vi "Sweep SL WL.vi"(8 "error in (no error)":errorcluster, 9 "Sweep outfile":path, 10 "addr":i32, 11 "instrument handle":refnum<k15>) -> (0 "error out":errorcluster, 1 "final current (A)":dbl, 2 "final resistance (ohm)":dbl, 3 "instrument handle out":refnum<k15>)   [LabVIEW 2018]
uses:
  <vilib>/Utility/file.llb/Write Delimited Spreadsheet (DBL).vi
panel:
  out "i":i32
  out "PW":i32
  out "SL voltage (V)":dbl
  out "WL voltage (V)":dbl
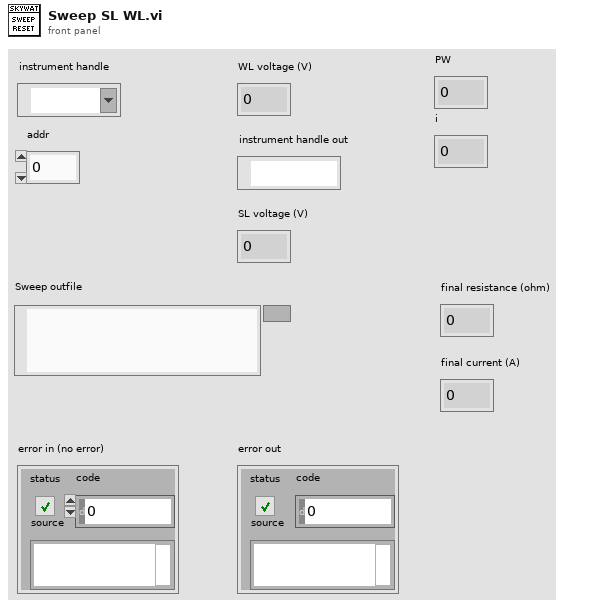
[diagram p1: front panel]
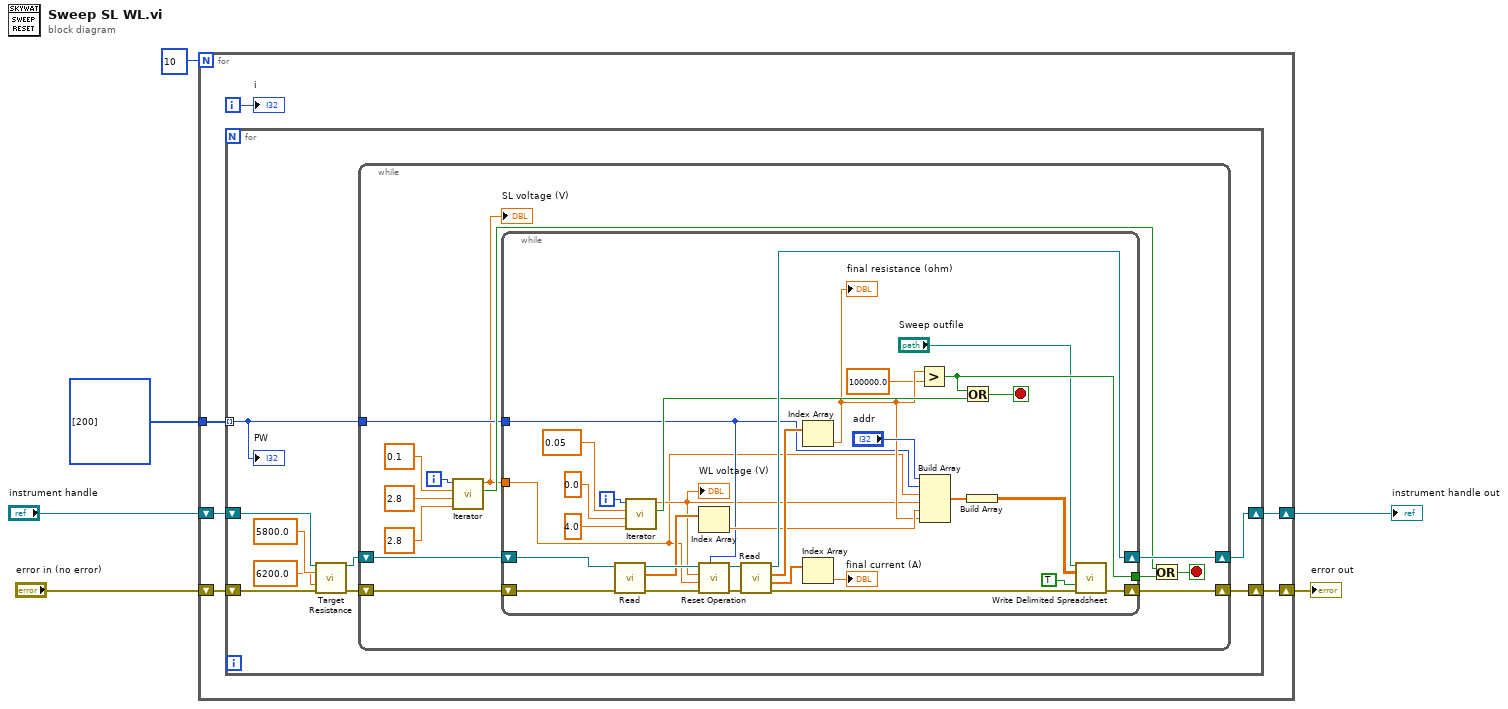
[diagram p0: block diagram]
diagram:
  n1 = for {
    N: 10 -> [_]
    tunnel: i32[] [200] -> [w8]
    shift-right: [w12] -> w6
    shift-left: "instrument handle" -> [w11]
    shift-right: [w9] -> w3
    shift-left: "error in (no error)" -> [w10]
    i -> [w7]
    n2 = for {
      shift-right: [w21] -> w12
      shift-left: w11 -> [w15]
      shift-right: [w20] -> w9
      shift-left: w10 -> [w16]
      tunnel: w8 -> [w19] mode=indexing
      n3 = call "Target Resistance.vi"("instrument handle"=w15, "Lower resistance (ohm)"=5800.0 ("Upper resistance (ohm)"), "Upper resistance (ohm)"=6200.0 ("Lower resistance (ohm)"), "error in (no error)"=w16) -> ("instrument handle out"=w14:refnum<k15>, "error out"=w13:errorcluster)  [unwired: 4 in, 6 out]
      n4 = while {
        shift-right: [w31] -> w21
        shift-left: w14 -> [w23]
        shift-right: [w30] -> w20
        shift-left: w13 -> [w22]
        tunnel: w19 -> [w26]
        i -> [w32]
        stop <- w27 stop-if-true
        n5 = call "Iterator.vi"("Final Value"=2.8 ("y"), "Initial Value"=2.8 ("y"), "Step"=0.1 ("x"), "i"=w32) -> ("End Loop"=w29:bool, "Current Value"=w25:dbl)  [unwired: 6 in]
        "SL voltage (V)" <- w25
        n6 = while {
          shift-right: [w55] -> w31
          shift-left: w23 -> [w38]
          shift-right: [w58] -> w30
          shift-left: w22 -> [w39]
          tunnel: w25 -> [w35]
          tunnel: w26 -> [w43]
          tunnel: [w46] -> w28
          i -> [w65]
          stop <- w50 stop-if-true
          n7 = call "Read.vi"("error in (no error)"=w39, "instrument handle"=w38) -> ("error out"=w40:errorcluster, "resistances (ohm)"=w37:dbl[], "instrument handle out"=w41:refnum<k15>)  [unwired: 6 in, 1 out]
          n8 = call "Iterator.vi"("Final Value"=4.0 ("y"), "Initial Value"=0.0 ("y"), "Step"=0.05 ("x"), "i"=w65) -> ("End Loop"=w49:bool, "Current Value"=w36:dbl)  [unwired: 6 in]
          "WL voltage (V)" <- w36
          n9 = Index Array(array=w37) -> (element=w51:dbl)  [unwired: 1 in]
          n10 = call "Reset Operation.vi"("PW"=w43, "error in (no error)"=w40, "SLV"=w35, "WLV"=w36, "instrument handle"=w41) -> ("error out"=w45:errorcluster, "instrument handle out"=w44:refnum<k15>)  [unwired: 5 in]
          n11 = call "Read.vi"("error in (no error)"=w45, "instrument handle"=w44) -> ("error out"=w56:errorcluster, "currents (A)"=w53:dbl[], "resistances (ohm)"=w54:dbl[], "instrument handle out"=w55:refnum<k15>)  [unwired: 6 in]
          n12 = Index Array(array=w54) -> (element=w48:dbl)  [unwired: 1 in]
          "final resistance (ohm)" <- w48
          n13 = Index Array(array=w53) -> (element=→"final current (A)":dbl)  [unwired: 1 in]
          n14 = Greater?(x=w48, y=100000.0 ("x")) -> (0:w46:bool)
          n15 = Build Array("addr", w43, w35, w36, w51, w48) -> (w60:dbl[])
          n16 = Or(x=w46, y=w49) -> (x .or. y?=w50:bool)
          n17 = Build Array(w60) -> (w61:dbl[][])
          n18 = call-poly <vilib>:"Write Delimited Spreadsheet.vi"("file path (dialog if empty)"="Sweep outfile", "2D data"=w61, "append to file? (new file:F)"=TRUE, "error in (no error)"=w56) -> ("error out"=w58:errorcluster)  [unwired: 10 in, 1 out]
        }
        n19 = Or(x=w29, y=w28) -> (x .or. y?=w27:bool)
      }
      "PW" <- w19
    }
    "i" <- w7
  }
  "error out" <- w3
  "instrument handle out" <- w6
